vi "FPGA_laser_task_test.vi"() -> ()   [LabVIEW 2015]
uses:
  <vilib>/rvi/eio/common/nirviEmuTemplateMethod_errors.vi
  <vilib>/eio/EIONode/EIONode.xnode
panel:
  in  "561 Laser Power":i16[](array[numeric])=[0, 0, 0, 0, 0]
  in  "N":i32=4
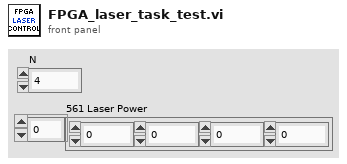
[diagram p1: front panel]
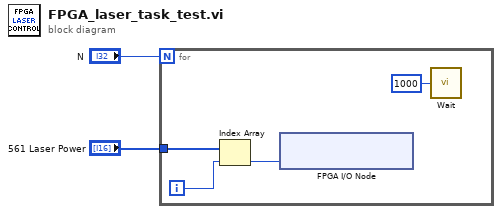
[diagram p0: block diagram]
diagram:
  n1 = for {
    N: "N" -> [_]
    tunnel: "561 Laser Power" -> [w6]
    i -> [w5]
    n2 = Index Array(array=w6, index=w5) -> (element=w4:i16)
    n3 = xnode "FPGA I/O Node"("Connector0/AO0"=w4) -> ()  [unwired: 1 in, 1 out]
    n4 = call "Wait"("Count(mSec)"=u32 1000) -> ()  [unwired: 1 out]
  }
